vi "DIO 1 Samples（Host）.vi"() -> ()   [LabVIEW 2019]
uses:
  <vilib>/FPGAPlugInAG/ELVIS III/niLvFpga_Open_ELVIS III.vi
  <vilib>/rvi/interface/common/dynamic/niFpgaDynamicAddResources.vi
  <vilib>/Utility/error.llb/Error Cluster From Error Code.vi
  <vilib>/rvi/errors/niLvFpgaAdjustHostInterfaceError.vi
  <vilib>/FPGAPlugInAG/Dynamic/niLvFpga_Close_Dynamic.vi
  <vilib>/rvi/interface/nirviOpenFPGA/nirviOpenFPGA.xnode
  FPGA Bitfiles/analogio-fpga_FPGATarget_DIO1Samples_iUXAejmrQ8c.lvbitx
  DIO 1 Samples.vi
  <vilib>/rvi/interface/nirviReadWriteControl/nirviReadWriteControl.xnode
  <vilib>/rvi/interface/nirviCloseFPGA/nirviCloseFPGA.xnode
  NiFpgaLv.dll
  <vilib>/rvi/interface/Simulation/niFpgaSimulationCallBeginRW.vi
panel:
  in  "停止":bool
  out "B.IN":bool[](array[boolean])
  out "A.IN":bool[](array[boolean])
  in  "B.DIR":bool[](array[boolean])
  in  "B.OUT":bool[](array[boolean])
  in  "A.OUT":bool[](array[boolean])
  in  "A.DIR":bool[](array[boolean])
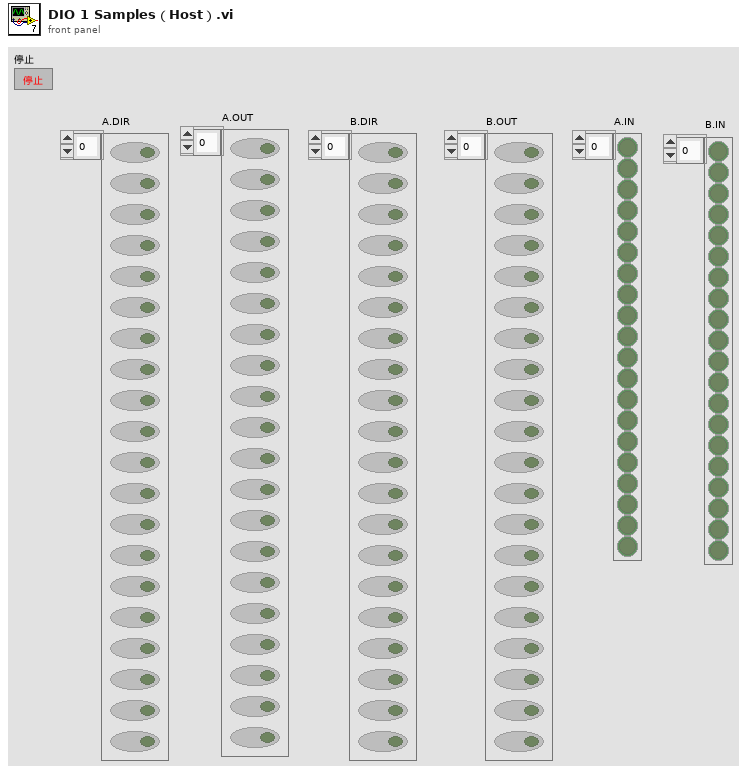
[diagram p1: front panel]
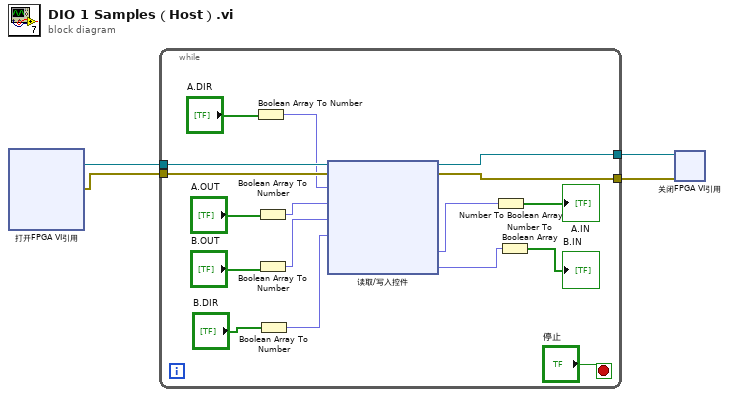
[diagram p0: block diagram]
diagram:
  n1 = xnode "打开FPGA VI引用"() -> ("FPGA VI引用输出"=w4:refnum<k20>, "错误输出"=w3:errorcluster)  [unwired: 2 in]
  n2 = while {
    tunnel: w4 -> [w21]
    tunnel: w3 -> [w20]
    tunnel: [w11] -> w2
    tunnel: [w10] -> w1
    stop <- "停止" stop-if-true
    n3 = Boolean Array To Number ("布尔数组至数值转换")(Boolean array="A.DIR") -> (number=w18:fxp<+,20,20>)
    n4 = Boolean Array To Number ("布尔数组至数值转换")(Boolean array="A.OUT") -> (number=w9:fxp<+,20,20>)
    n5 = Boolean Array To Number ("布尔数组至数值转换")(Boolean array="B.OUT") -> (number=w8:fxp<+,20,20>)
    n6 = Boolean Array To Number ("布尔数组至数值转换")(Boolean array="B.DIR") -> (number=w7:fxp<+,20,20>)
    n7 = xnode "读取/写入控件"("FPGA VI引用输入"=w21, "错误输入"=w20, "DIO.A_19:0.DIR"=w18, "DIO.A_19:0.OUT"=w9, "DIO.B_19:0.OUT"=w8, "DIO.B_19:0.DIR"=w7) -> ("FPGA VI引用输出"=w10:refnum<k20>, "错误输出"=w11:errorcluster, "DIO.A_19:0.IN"=w6:fxp<+,20,20>, "DIO.B_19:0.IN"=w5:fxp<+,20,20>)
    n8 = Number To Boolean Array(number=w6) -> (Boolean array=→"A.IN":bool[])
    n9 = Number To Boolean Array(number=w5) -> (Boolean array=→"B.IN":bool[])
  }
  n10 = xnode "关闭FPGA VI引用"("FPGA VI引用输入"=w1, "错误输入"=w2) -> ()  [unwired: 1 out]
